vi "ConnectorPaneSettings.vi"() -> ()   [LabVIEW 2020]
doc: "Example of using options of connectors in subVI. Comments in Polish."
uses:
  <vilib>/Instr/_visa.llb/VISA Configure Serial Port (Instr).vi
panel:
  in  "Coefficient(1)":dbl=1.0
  out "Result":dbl
  out "Error Out":errorcluster
  in  "Error In":errorcluster
  in  "Main value":dbl format="%#_13g"
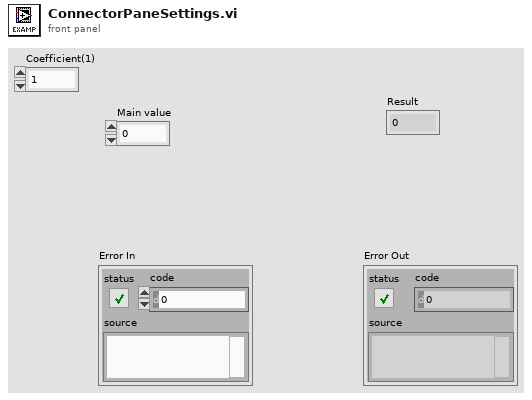
[diagram p1: front panel]
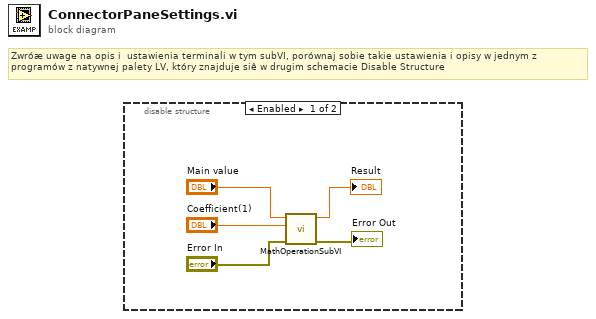
[diagram p0: block diagram]
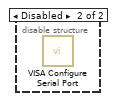
[diagram p2: hidden frame]
diagram:
  # "Zwróæ uwage na opis i  ustawienia terminali w tym subVI, porównaj sobie takie ustawienia i opisy w jednym z \nprogramów z natywnej palety LV, który znajduje siê w drugim schemacie Disable Structure"
  n1 = disable-structure shown="Enabled" {
    frame Enabled {
      n2 = call "MathOperationSubVI.vi"("Error In"="Error In", "Coefficient(1)"="Coefficient(1)", "Main value in"="Main value") -> ("Error Out"=→"Error Out":errorcluster, "Result"=→"Result":dbl)  [unwired: 7 in]
    }
    frame Disabled {
      n3 = call-poly "VISA Configure Serial Port"() -> ()  [unwired: 14 in, 2 out]
    }
  }
